vi "Get Controller Rate.vi"(8 "error in (no error)":errorcluster, 11 "Device Reference In":T1=18446744073709551615 format="%.0x") -> (0 "error out":errorcluster, 2 "System dt in uS":u32, 3 "System dt in Secs":dbl)   [LabVIEW 2010, in "NI PXI-4072 DMM Custom Device.lvlib"]
uses:
  <vilib>/NI VeriStand/Custom Device API/Custom Device Item Ref.ctl
  NI PXI-4072 DMM Custom Device.lvlib
  <vilib>/NI Veristand/Custom Device Tools/Custom Device Utility Library/Custom Device Utility Library.lvlib
  <vilib>/NI Veristand/Custom Device API/Custom Device API.lvlib
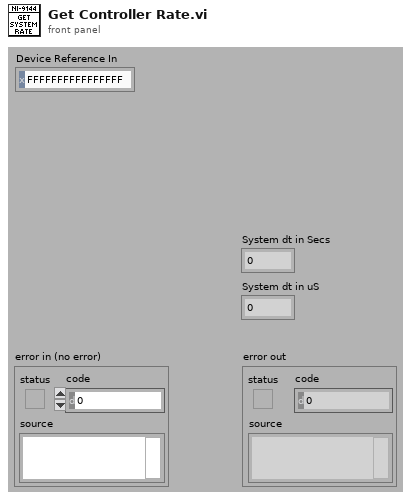
[diagram p1: front panel]
types:
  T1 = typedef "Custom Device API.lvlib/Custom Device Item Ref.ctl" = u64
  T2 = typedef "Custom Device API.lvlib/Custom Device Channel.ctl" = cluster{"Type":T3, "Units":string, "Default Value":dbl, "Faultable":bool, "Scalable":bool}
  T3 = typedef "Custom Device API.lvlib/Custom Device Channel Type.ctl" = enum16{"Input", "Output"}
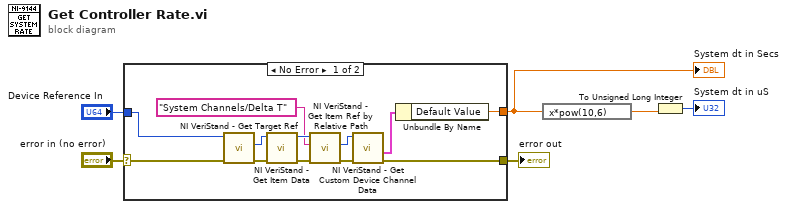
[diagram p0: block diagram]
diagram:
  n1 = case shown="No Error" "error in (no error)" {
    selector: "error in (no error)" -> [w7 w19]
    tunnel: [w10 w19] -> w6
    tunnel: "Device Reference In" -> [w8 _]
    tunnel: [w9 _] -> w2
    frame No Error {
      n2 = call <vilib>:"NI VeriStand - Get Target Ref.vi"("error in"=w7, "Item Ref in"=w8) -> ("error out"=w17:errorcluster, "Target Ref"=w18:T1)  [unwired: 8 out]
      n3 = call <vilib>:"NI VeriStand - Get Item Data.vi"("error in (no error)"=w17, "Item Ref in"=w18) -> ("error out"=w15:errorcluster, "Item Ref out"=w16:T1)  [unwired: 8 out]
      n4 = call <vilib>:"NI VeriStand - Get Item Ref by Relative Path.vi"("error in"=w15, "Relative Item Path"="System Channels/Delta T", "Section Ref in"=w16) -> ("error out"=w12:errorcluster, "Item Ref"=w13:T1)  [unwired: 7 out]
      n5 = call <vilib>:"NI VeriStand - Get Custom Device Channel Data.vi"("error in (no error)"=w12, "Channel Ref in"=w13) -> ("error out"=w10:errorcluster, "Channel"=w11:T2)  [unwired: 8 out]
      n6 = Unbundle By Name(w11) -> ("Default Value"=w9:dbl)
    }
    frame Error {
    }
  }
  "error out" <- w6
  "System dt in Secs" <- w2
  n7 = expression code="x*pow(10,6)"(w2) -> (w1:dbl)
  n8 = To Unsigned Long Integer(number=w1) -> (unsigned 32bit integer=→"System dt in uS":u32)
